vi "Save Front Panel controls to cfg file.vi"(7 "error in":errorcluster, 9 "UI element":T1, 10 "VI reference":refnum<vi>) -> (0 "error out":errorcluster, 3 "VI reference out":refnum<vi>)   [LabVIEW 2013]
doc: "This .vi saves the flattened control values to file."
uses:
  User interface config file selector enum.ctl
  HHMI - Config file functional global mode enum.ctl
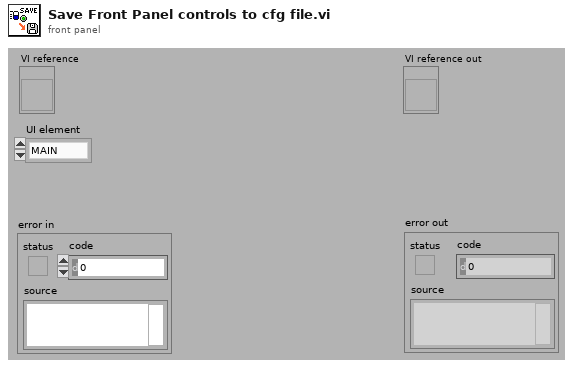
[diagram p1: front panel]
types:
  T1 = typedef "User interface config file selector enum.ctl" = enum16{"MAIN"}
  T2 = typedef "HHMI - Config file functional global mode enum.ctl" = enum16{"Set Filepath", "Read file", "Rewrite file"}
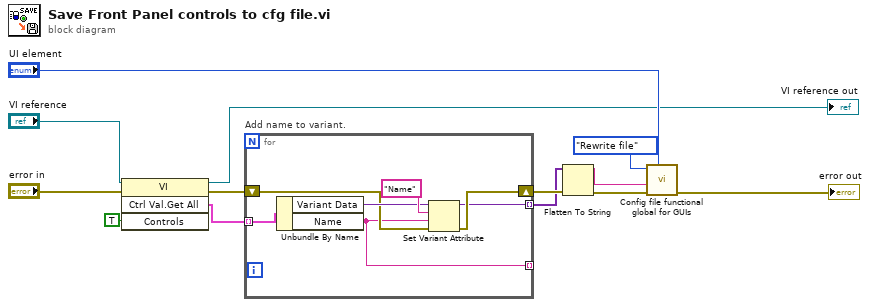
[diagram p0: block diagram]
diagram:
  n1 = invoke class="VI" method="Ctrl Val.Get All"(reference="VI reference", error in="error in", "Controls"=TRUE) -> (reference out=→"VI reference out":refnum<vi>, error out=w10:errorcluster, "Get All Control Values Variant"=w11:cluster{"Name":string, "Variant Data":variant}[])  [unwired: 1 in, 1 out]
  n2 = for "Add name to variant." {
    tunnel: w11 -> [w20] mode=indexing
    shift-right: [w16] -> w9
    shift-left: w10 -> [w17]
    tunnel: [w15] -> w8 mode=indexing
    tunnel: [w14] -> _ mode=indexing
    n3 = Unbundle By Name(w20) -> ("Variant Data"=w18:variant, "Name"=w14:string)
    n4 = Set Variant Attribute(Variant=w18, name="Name", value=w14, error in=w17) -> (Variant out=w15:variant, error out=w16:errorcluster)  [unwired: 1 out]
  }
  n5 = Flatten To String(anything=w8, error in (no error)=w9) -> (data string=w5:string, error out=w7:errorcluster)  [unwired: 3 out]
  n6 = call "Config file functional global for GUIs.vi"("GUI elements"="UI element", "error in"=w7, "text to write"=w5, "Mode"=HHMI_-_Config_file_functional_global_mode_enum."Rewrite file") -> ("error out"=→"error out":errorcluster)  [unwired: 1 in, 6 out]
